vi "US_two_Wire.vi"(7 "start ping":bool, 9 "Timeout (usec)":u16, 10 "Echo_Line":refnum<k21>, 11 "Ping_Line":refnum<k21>) -> (1 "echo_time(us)":u16, 2 "busy":bool)   [LabVIEW 2019]
uses:
  us_state.ctl
  <vilib>/rvi/Emulation/niFpgaGetClockAttributes.vi
  <vilib>/rvi/Emulation/niFpgaSctlEmulationGetInTimedLoop.vi
  <vilib>/rvi/Emulation/niFpgaEmulationReportErrorSimple.vi
  <vilib>/rvi/eio/common/nirviEmuTemplateMethod_errors.vi
  <vilib>/rvi/Emulation/niFpgaCriticalErrorInLSC.vi
  <vilib>/eio/EIONode/EIONode.xnode
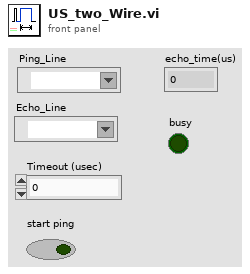
[diagram p1: front panel]
types:
  T1 = typedef "us_state.ctl" = enum16{"idle", "ping", "set_to_input", "hold_off", "listen"}
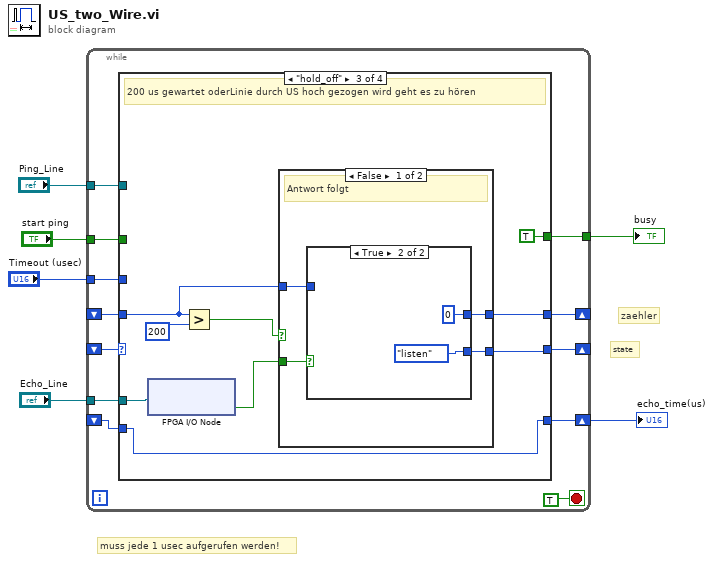
[diagram p0: block diagram]
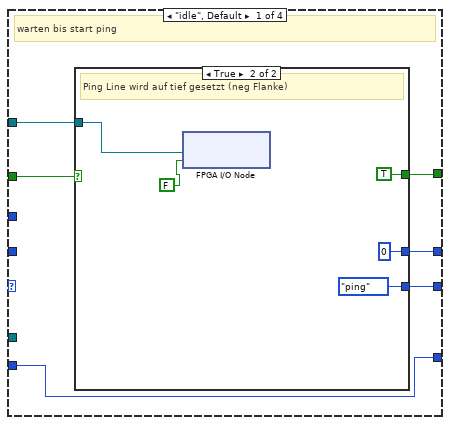
[diagram p2: hidden frame]
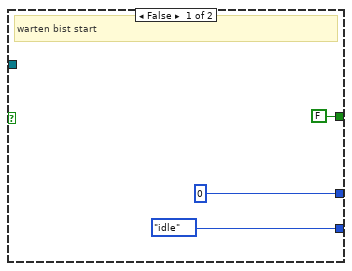
[diagram p3: hidden frame]
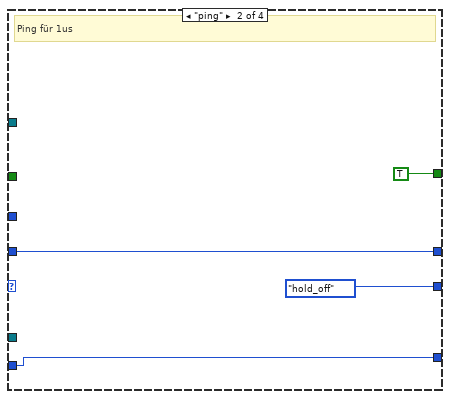
[diagram p4: hidden frame]
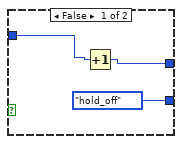
[diagram p5: hidden frame]
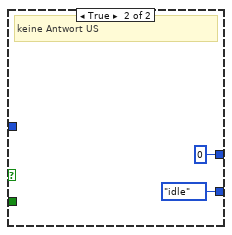
[diagram p6: hidden frame]
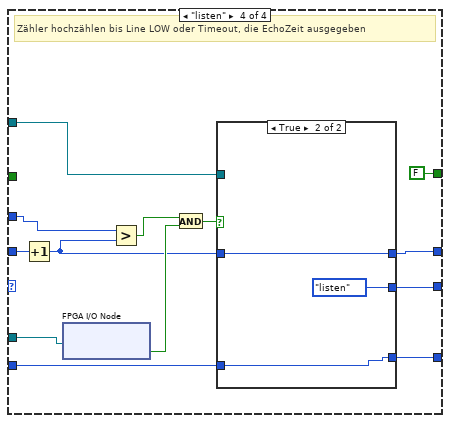
[diagram p7: hidden frame]
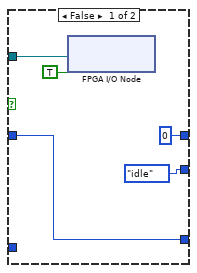
[diagram p8: hidden frame]
diagram:
  # "muss jede 1 usec aufgerufen werden!"
  # "zaehler"
  # "state"
  n1 = while {
    shift-right: [w16] -> _
    shift-left: _ -> [w13]
    tunnel: "Ping_Line" -> [w18]
    shift-right: [w14] -> _
    shift-left: _ -> [w17]
    tunnel: "Timeout (usec)" -> [w12]
    tunnel: "start ping" -> [w11]
    tunnel: [w10] -> w3
    tunnel: "Echo_Line" -> [w9]
    shift-right: [w8] -> w1
    shift-left: _ -> [w7]
    stop <- TRUE stop-if-true
    n2 = case shown="\"hold_off\"" w17 {
      tunnel: w18 -> [w24 _ _ w59]
      tunnel: [w23 w36 w43 w64] -> w16
      tunnel: [w22 us_state."hold_off" w42 w62] -> w14
      tunnel: w13 -> [_ w36 w44 w69]
      tunnel: w12 -> [_ _ _ w68]
      tunnel: w11 -> [w21 _ _ _]
      tunnel: [w20 TRUE TRUE FALSE] -> w10
      tunnel: w9 -> [_ _ w38 w61]
      tunnel: [w19 w33 w37 w58] -> w8
      tunnel: w7 -> [w19 w33 w37 w57]
      frame "idle", Default {
        # "warten bis start ping"
        n3 = case shown="True" w21 {
          tunnel: w24 -> [_ w30]
          tunnel: [u16 0 u16 0] -> w23
          tunnel: [us_state."idle" us_state."ping"] -> w22
          tunnel: [FALSE TRUE] -> w20
          frame False {
            # "warten bist start"
          }
          frame True {
            # "Ping Line wird auf tief gesetzt (neg Flanke)"
            n4 = xnode "FPGA I/O Node"("I/O Item"=FALSE, "FPGA I/O In"=w30) -> ()  [unwired: 1 out]
          }
        }
      }
      frame "ping" {
        # "Ping für 1us"
      }
      frame "hold_off" {
        # "200 us gewartet oderLinie durch US hoch gezogen wird geht es zu hören"
        n5 = xnode "FPGA I/O Node"("FPGA I/O In"=w38) -> ("I/O Item"=w41:bool)  [unwired: 1 out]
        n6 = Greater?(x=w44, y=u16 200) -> (0:w39:bool)
        n7 = case shown="False" w39 {
          tunnel: w44 -> [w49 _]
          tunnel: [w48 u16 0] -> w43
          tunnel: [w47 us_state."idle"] -> w42
          tunnel: w41 -> [w46 _]
          frame False {
            # "Antwort folgt"
            n8 = case shown="True" w46 {
              tunnel: w49 -> [w52 _]
              tunnel: [w51 u16 0] -> w48
              tunnel: [us_state."hold_off" us_state."listen"] -> w47
              frame False {
                n9 = Increment(x=w52) -> (x+1=w51:u16)
              }
              frame True {
              }
            }
          }
          frame True {
            # "keine Antwort US"
          }
        }
      }
      frame "listen" {
        # "Zähler hochzählen bis Line LOW oder Timeout, die EchoZeit ausgegeben"
        n10 = Increment(x=w69) -> (x+1=w63:u16)
        n11 = xnode "FPGA I/O Node"("FPGA I/O In"=w61) -> ("I/O Item"=w65:bool)  [unwired: 1 out]
        n12 = Greater?(x=w68, y=w63) -> (0:w66:bool)
        n13 = And(x=w66, y=w65) -> (x .and. y?=w67:bool)
        n14 = case shown="True" w67 {
          tunnel: [u16 0 w77] -> w64
          tunnel: w63 -> [w70 w77]
          tunnel: [us_state."idle" us_state."listen"] -> w62
          tunnel: w59 -> [w72 _]
          tunnel: [w70 w75] -> w58
          tunnel: w57 -> [_ w75]
          frame False {
            n15 = xnode "FPGA I/O Node"("I/O Item"=TRUE, "FPGA I/O In"=w72) -> ()  [unwired: 1 out]
          }
          frame True {
          }
        }
      }
    }
  }
  "busy" <- w3
  "echo_time(us)" <- w1
